vi "List Groups.vi"(8 "error in (no error)":errorcluster, 11 "Blackboard in":refnum<class "Blackboard.lvclass">) -> (0 "error out":errorcluster, 2 "Groups":string[](array[string]), 3 "Blackboard out":refnum<class "Blackboard.lvclass">)   [LabVIEW 2021, in "Blackboard.lvclass"]
uses:
  Blackboard.lvclass
  Blackboard.lvclass/Blackboard.ctl
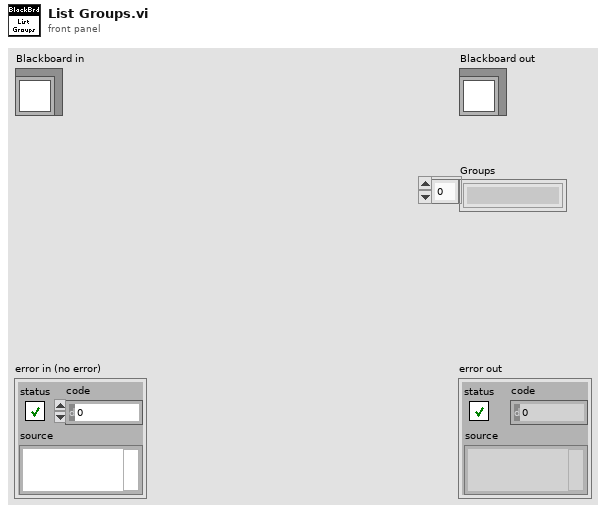
[diagram p1: front panel]
types:
  T1 = typedef "Blackboard.lvclass/Groups Type.ctl" = cluster{"Data":T2[], "Map":T5}
  T2 = typedef "Blackboard.lvclass/Data DVR Type.ctl" = cluster{"Tags":T3, "Data Refs":T4}
  T3 = typedef "Blackboard.lvclass/Tags Map Type.ctl" = map{string, refnum<class "Abs_Value.lvclass">}
  T4 = typedef "Local Bus.lvclass/Data Value References.ctl" = cluster{"Boolean":refnum<data-value>, "String":refnum<data-value>, "DBL":refnum<data-value>, "SGL":refnum<data-value>, "EXT":refnum<data-value>, "U8":refnum<data-value>, "U16":refnum<data-value>, "U32":refnum<data-value>, "U64":refnum<data-value>, "I8":refnum<data-value>, "I16":refnum<data-value>, "I32":refnum<data-value>, "I64":refnum<data-value>, "CDBL":refnum<data-value>, "CSGL":refnum<data-value>, "CEXT":refnum<data-value>, "Time":refnum<data-value>, "Variant":refnum<data-value>, "Waveform":refnum<data-value>, "Type":refnum<data-value>}
  T5 = typedef "Blackboard.lvclass/Group Map Type.ctl" = map{string, i32}
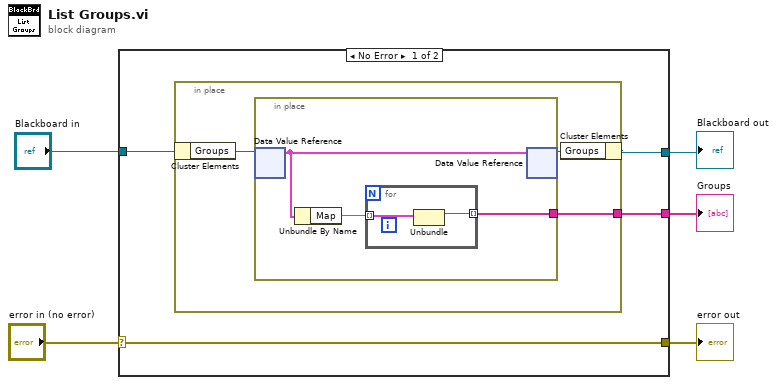
[diagram p0: block diagram]
diagram:
  n1 = case shown="No Error" "error in (no error)" {
    selector: "error in (no error)" -> [w7 w19]
    tunnel: [w7 w19] -> w3
    tunnel: [w9 w18] -> w2
    tunnel: "Blackboard in" -> [w8 w18]
    tunnel: [w6 _] -> w1
    frame No Error {
      n2 = in-place {
        in-place-border: [w10] -> w6
        n3 = in-place-cluster #1(w8) -> ("Groups"=w12:refnum<data-value>)
        n4 = in-place {
          in-place-border: [w13] -> w10
          n5 = in-place-dvr #2(w12) -> (w15:T1)  [unwired: 1 out]
          n6 = Unbundle By Name(w15) -> ("Map"=w14:T5)
          n7 = for {
            tunnel: w14 -> [w17] mode=indexing
            tunnel: [w16] -> w13 mode=indexing
            n8 = Unbundle(w17) -> (w16:string)  [unwired: 1 out]
          }
          n9 = in-place-dvr #2(w15) -> (w11:refnum<data-value>)  [unwired: 1 out]
        }
        n10 = in-place-cluster #1("Groups"=w11) -> (w9:refnum<class "Blackboard.lvclass">)
      }
    }
    frame Error {
    }
  }
  "error out" <- w3
  "Blackboard out" <- w2
  "Groups" <- w1
